vi "Sound Probe.vi"(11 "Sound.lvclass":refnum<class "Sound.lvclass">) -> (2 "Value String":string, 3 "Boolean":bool)   [LabVIEW 2010, in "Sound.lvclass"]
uses:
  Sound.lvclass
panel:
  out "Waveforms":waveform(dbl)[](graph)
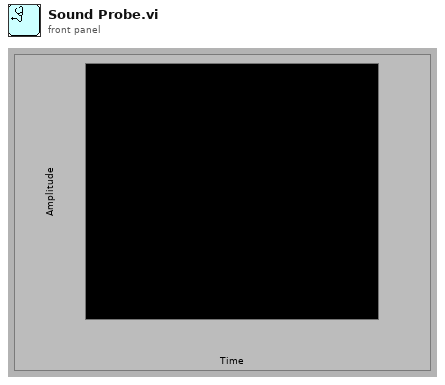
[diagram p1: front panel]
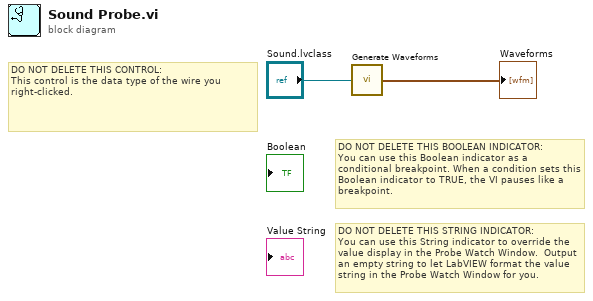
[diagram p0: block diagram]
diagram:
  # "DO NOT DELETE THIS STRING INDICATOR: \nYou can use this String indicator to override the value display in the Probe Watch Window.  Output an empty string to let LabVIEW format the value string in the Probe Watch Window for you."
  # "DO NOT DELETE THIS BOOLEAN INDICATOR: \nYou can use this Boolean indicator as a conditional breakpoint. When a condition sets this Boolean indicator to TRUE, the VI pauses like a breakpoint."
  # "DO NOT DELETE THIS CONTROL: \nThis control is the data type of the wire you right-clicked."
  n1 = call-dynamic "Generate Waveforms.vi"("Sound.lvclass"="Sound.lvclass") -> ("Waveforms"=→"Waveforms":waveform(dbl)[])
